vi "Station1_Data_Log.vi"(8 "error in (no error)":errorcluster, 11 "Cluster":T2) -> (0 "error out":errorcluster, 3 "Array":string[](array[string]))   [LabVIEW 2017]
uses:
  <vilib>/addons/database/Connection.llb/Conn ObjectReference.ctl
  <vilib>/addons/database/NI_Database_API.lvlib
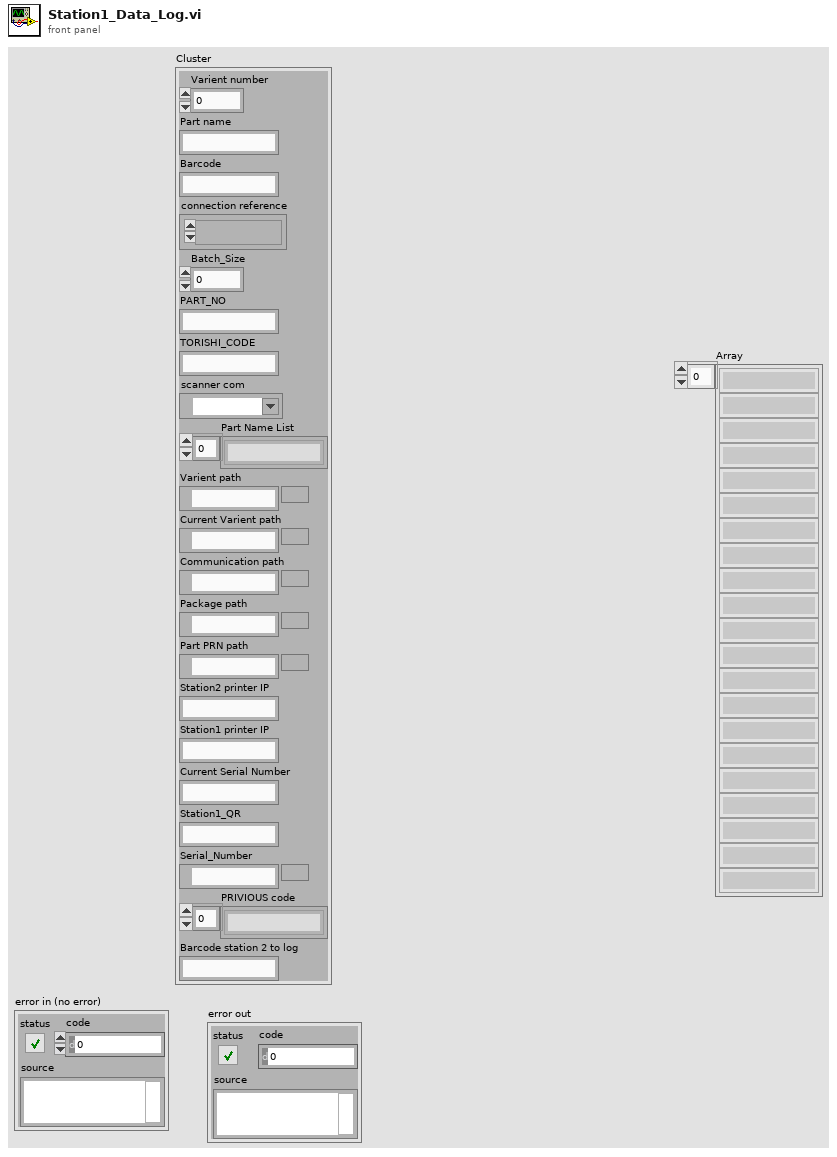
[diagram p1: front panel]
types:
  T1 = typedef "NI_Database_API.lvlib/Conn ObjectReference.ctl" = refnum<k1>
  T2 = cluster{"Varient number":u16, "Part name":string, "Barcode":string, "connection reference":T1, "Batch_Size":u16, "PART_NO":string, "TORISHI_CODE":string, "scanner com":refnum<visa-resource-name>, "Part Name List":string[], "Varient path":path, "Current Varient path":path, "Communication path":path, "Package path":path, "Part PRN path":path, "Station2 printer IP":string, "Station1 printer IP":string, "Current Serial Number":string, "Station1_QR":string, "Serial_Number":path, "PRIVIOUS code":string[], "Barcode station 2 to log":string}
  T3 = cluster{"date/time string":string, "date/time string":string, string, "Part name":string, "PART_NO":string, "TORISHI_CODE":string, "Shift":string, string, "station1 rst":string, string, "result string":string, "Station1_QR":string, string, string, string, string, string, string, string, string, string}
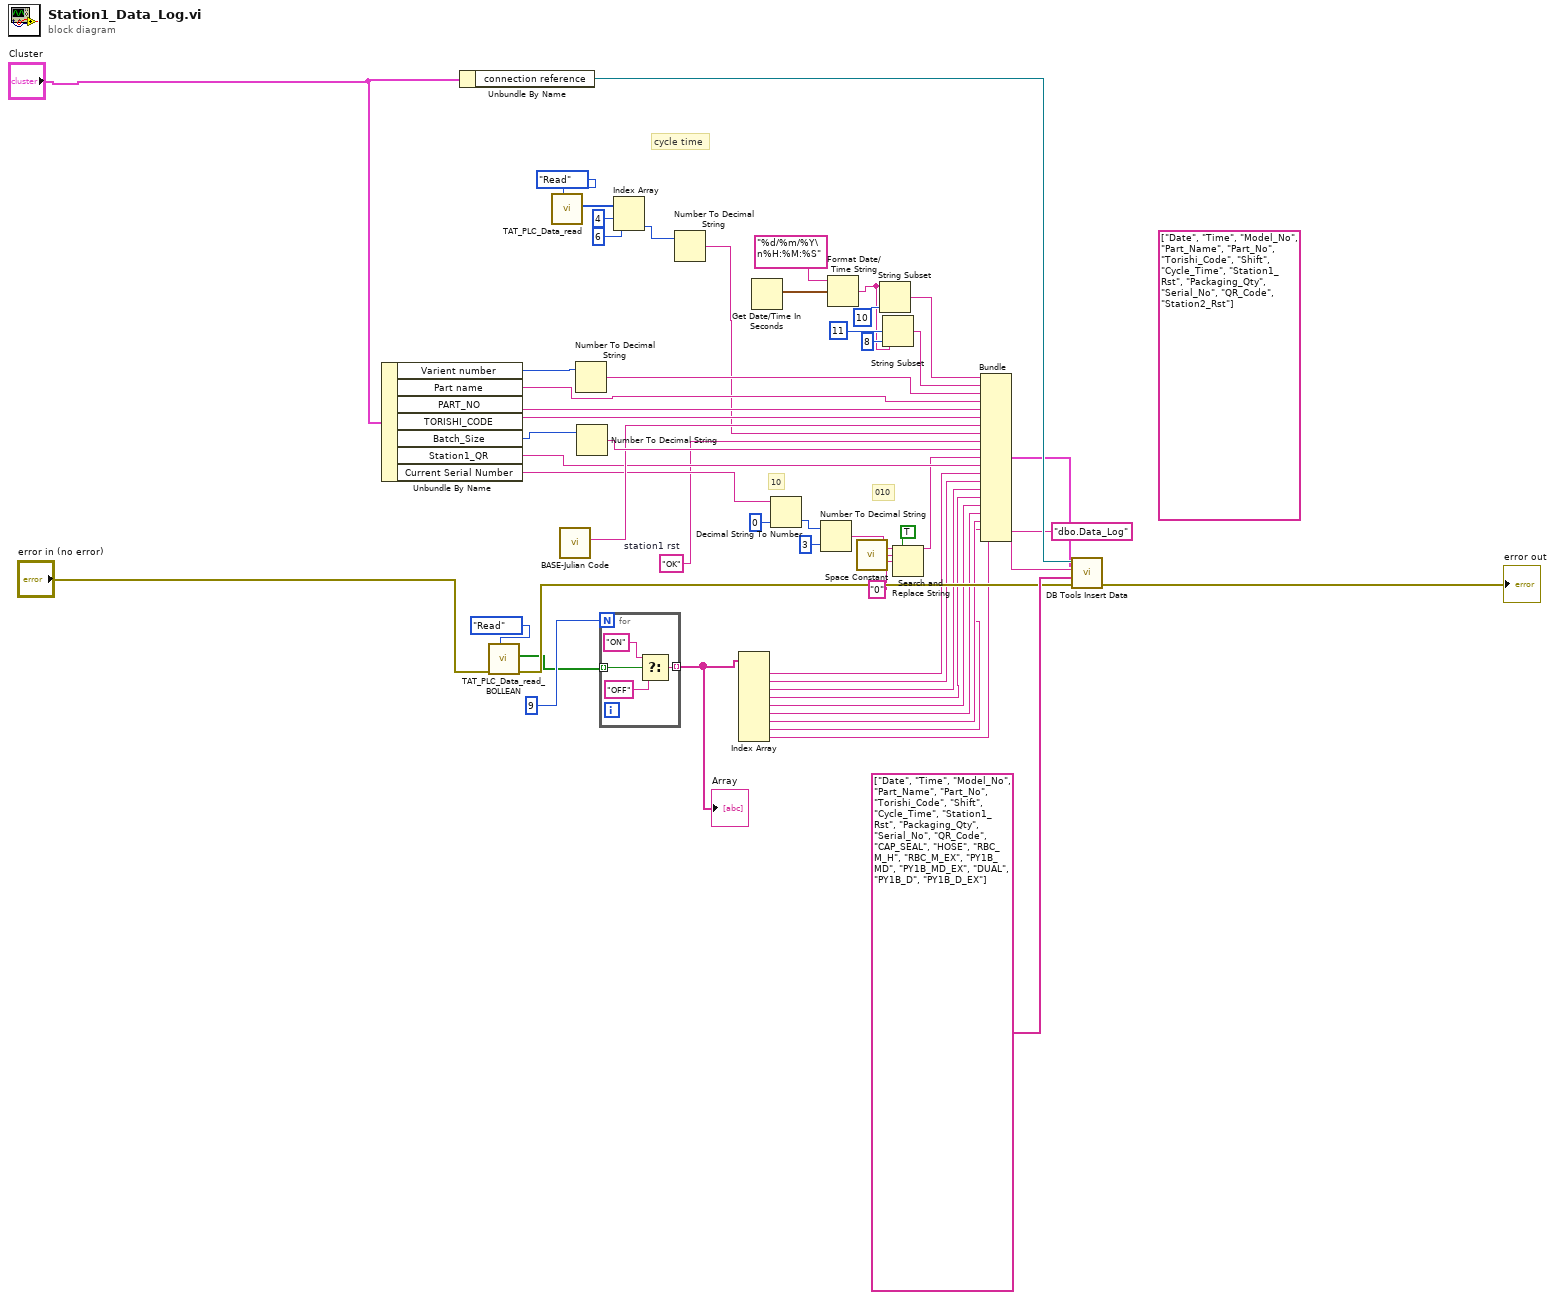
[diagram p0: block diagram]
diagram:
  w14 = "OK"  # station1 rst
  (unwired) string[] ["Date", "Time", "Model_No", "Part_Name", "Part_No", "Torishi_Code", "Shift", "Cycle_Time", "Station1_Rst", "Packaging_Qty", "Serial_No", "QR_Code", "Station2_Rst"] ("columns 2")
  # "010"
  # "10"
  # "cycle time"
  n1 = Unbundle By Name("Cluster") -> ("Varient number"=w48:u16, "Part name"=w50:string, "PART_NO"=w51:string, "TORISHI_CODE"=w52:string, "Batch_Size"=w53:u16, "Station1_QR"=w24:string, "Current Serial Number"=w16:string)
  n2 = Unbundle By Name("Cluster") -> ("connection reference"=w35:T1)
  n3 = call "TAT_PLC_Data_read_BOLLEAN.vi"("Enum"=enum16{"Read", "Write"}."Read", "error in (no error)"="error in (no error)") -> ("error out"=w37:errorcluster, "Array 2"=w11:bool[])  [unwired: 8 in]
  n4 = call "TAT_PLC_Data_read.vi"("Enum"=enum16{"Read", "Write"}."Read") -> ("Array 2"=w30:u16[])  [unwired: 9 in, 1 out]
  n5 = call "BASE-Julian Code.vi"() -> ("Shift"=w31:string)  [unwired: 6 in, 5 out]
  n6 = Number To Decimal String(number=w48) -> (decimal integer string=w49:string)  [unwired: 1 in]
  n7 = Number To Decimal String(number=w53) -> (decimal integer string=w54:string)  [unwired: 1 in]
  n8 = for {
    N: 9 ("index") -> [_]
    tunnel: w11 -> [w58] mode=indexing
    tunnel: [w55] -> w10 mode=indexing
    n9 = Select(t="ON", s=w58, f="OFF") -> (s? t:f=w55:string)
  }
  "Array" <- w10
  n10 = Index Array(array=w30, index #1=4 ("index"), index #2=6 ("index")) -> (element #2=w26:u16)  [unwired: 1 out]
  n11 = Number To Decimal String(number=w26) -> (decimal integer string=w25:string)  [unwired: 1 in]
  n12 = Index Array(array=w10) -> (element #1=w9:string, element #2=w8:string, element #3=w7:string, element #4=w6:string, element #5=w5:string, element #6=w4:string, element #7=w3:string, element #8=w2:string, element #9=w1:string)  [unwired: 9 in]
  n13 = Get Date/Time In Seconds() -> (seconds since 1Jan1904=w40:timestamp)
  n14 = Decimal String To Number(string=w16, default (0L)=0 ("default (0 I32)")) -> (number=w22:i32)  [unwired: 1 in, 1 out]
  n15 = Number To Decimal String(number=w22, width (-)=i16 3) -> (decimal integer string=w20:string)
  n16 = Format Date/Time String(time format string (%c)="%d/%m/%Y\n%H:%M:%S", seconds (now)=w40) -> (date/time string=w42:string)  [unwired: 1 in]
  n17 = call <vilib>:"Space Constant.vi"() -> ("String"=w19:string)
  n18 = String Subset(string=w42, length (rest)=10 ("length (rest)")) -> (substring=w46:string)  [unwired: 1 in]
  n19 = String Subset(string=w42, offset (0)=11 ("length (rest)"), length (rest)=8 ("length (rest)")) -> (substring=w47:string)
  n20 = Search and Replace String(replace all?=TRUE ("replace all? (F)"), input string=w20, search string=w19, replace string="0" ("replace string (\"\")")) -> (result string=w15:string)  [unwired: 4 in, 3 out]
  n21 = Bundle("date/time string"=w46, "date/time string"=w47, w49, "Part name"=w50, "PART_NO"=w51, "TORISHI_CODE"=w52, "Shift"=w31, w25, "station1 rst"=w14, w54, "result string"=w15, "Station1_QR"=w24, w9, w8, w7, w6, w5, w4, w3, w2, w1) -> (w33:T3)  [unwired: 1 in]
  n22 = call <vilib>:"DB Tools Insert Data.vi"("data"=w33, "error in (no error)"=w37, "columns"=string[] ["Date", "Time", "Model_No", "Part_Name", "Part_No", "Torishi_Code", "Shift", "Cycle_Time", "Station1_Rst", "Packaging_Qty", "Serial_No", "QR_Code", "CAP_SEAL", "HOSE", "RBC_M_H", "RBC_M_EX", "PY1B_MD", "PY1B_MD_EX", "DUAL", "PY1B_D", "PY1B_D_EX"] ("columns 2"), "table"="dbo.Data_Log", "connection reference"=w35) -> ("error out"=→"error out":errorcluster)  [unwired: 5 in, 1 out]
